vi "sha256_scram_client_final.vi"(9 "password":string, 10 "server_first_message":string, 11 "client_first_message":string) -> (3 "client_final_message":string)   [LabVIEW 2019, in "hashlib.lvlib"]
doc: "Calculates the <b>SCRAM-SHA-256 FINAL CLIENT MESSAGE</b> to send to the server to validate authentication based on the <b>client_first_message</b>, the <b>server_first_message</b> and the original <b>password</b>.\n\nRFC 5802\n\nCreated by: Ryan Pacini"
uses:
  hashlib.lvlib
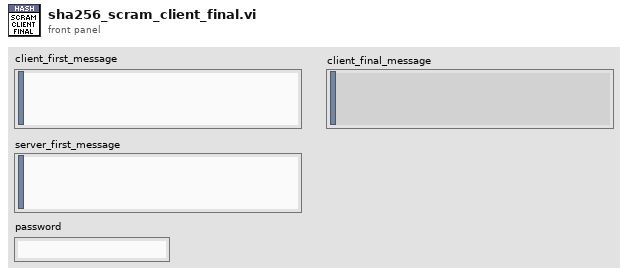
[diagram p1: front panel]
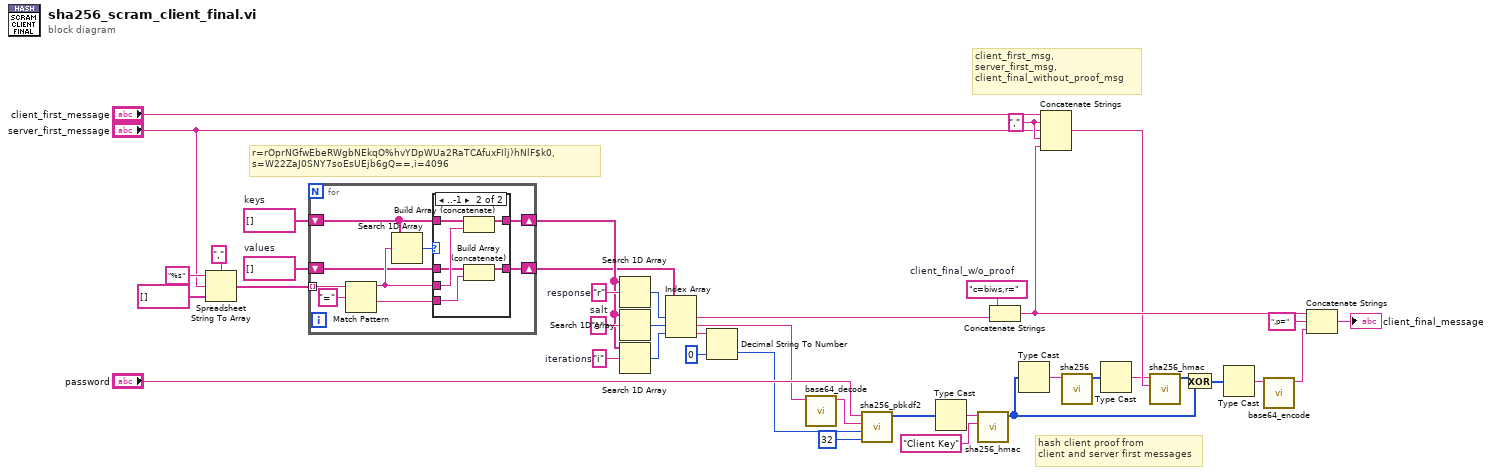
[diagram p0: block diagram]
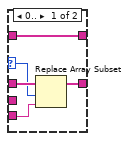
[diagram p2: hidden frame]
diagram:
  w3 = string[] []  # values
  w4 = string[] []  # keys
  w13 = "i"  # iterations
  w16 = "s"  # salt
  w17 = "r"  # response
  w34 = "," ("string")
  w33 = "c=biws,r="  # client_final_w/o_proof
  # "r=rOprNGfwEbeRWgbNEkqO%hvYDpWUa2RaTCAfuxFIlj)hNlF$k0,\ns=W22ZaJ0SNY7soEsUEjb6gQ==,i=4096"
  # "hash client proof from \nclient and server first messages"
  # "client_first_msg,\nserver_first_msg,\nclient_final_without_proof_msg"
  n1 = Spreadsheet String To Array(delimiter (Tab)=",", format string="%s", spreadsheet string="server_first_message", array type (2D Dbl)=string[] []) -> (array=w18:string[])
  n2 = for {
    tunnel: w18 -> [w50] mode=indexing
    shift-right: [w47] -> w2
    shift-left: w4 -> [w48]
    shift-right: [w43] -> w1
    shift-left: w3 -> [w44]
    n3 = Match Pattern(string=w50, regular expression="=") -> (before substring=w46:string, after substring=w42:string)  [unwired: 1 in, 2 out]
    n4 = Search 1D Array(1D array=w48, element=w46) -> (index of element=w45:i32)  [unwired: 1 in]
    n5 = case shown="..-1" w45 {
      selector: w45 -> [w52 _]
      tunnel: w48 -> [w55 w61]
      tunnel: [w55 w60] -> w47
      tunnel: w46 -> [_ w59]
      tunnel: w44 -> [w54 w58]
      tunnel: [w53 w57] -> w43
      tunnel: w42 -> [w51 w56]
      frame 0.. {
        n6 = Replace Array Subset(array=w54, new element=w51, index=w52) -> (w53:string[])
      }
      frame ..-1 {
        n7 = Build Array (concatenate)(w61, w59) -> (w60:string[])
        n8 = Build Array (concatenate)(w58, w56) -> (w57:string[])
      }
    }
  }
  n9 = Search 1D Array(1D array=w2, element=w17) -> (index of element=w15:i32)  [unwired: 1 in]
  n10 = Search 1D Array(1D array=w2, element=w16) -> (index of element=w14:i32)  [unwired: 1 in]
  n11 = Search 1D Array(1D array=w2, element=w13) -> (index of element=w12:i32)  [unwired: 1 in]
  n12 = Index Array(array=w1, index #1=w15, index #2=w14, index #3=w12) -> (element #1=w8:string, element #2=w7:string, element #3=w11:string)
  n13 = Decimal String To Number(string=w11, default (0L)=0 ("default (0 I32)")) -> (number=w6:i32)  [unwired: 1 in, 1 out]
  n14 = call "base64_decode.vi"("base64"=w7) -> ("string"=w21:string)  [unwired: 10 in]
  n15 = call "sha256_pbkdf2.vi"("dkLen (32octets=sha256)"=32 ("32octets=sha256"), "iterations"=w6, "salt"=w21, "password"="password") -> ("sha-256"=w29:u32[])  [unwired: 7 in]
  n16 = Type Cast(x=w29) -> (*(type *) &x=w31:string)  [unwired: 1 in]
  n17 = call "sha256_hmac.vi"("data"="Client Key" ("key"), "key"=w31) -> ("sha256"=w25:u32[])  [unwired: 9 in]
  n18 = Concatenate Strings(w33, w8) -> (w38:string)
  n19 = Type Cast(x=w25) -> (*(type *) &x=w22:string)  [unwired: 1 in]
  n20 = Concatenate Strings("client_first_message", w34, "server_first_message", w34, w38) -> (w35:string)
  n21 = call "sha256.vi"("data"=w22) -> ("sha256"=w23:u32[])  [unwired: 10 in]
  n22 = Type Cast(x=w23) -> (*(type *) &x=w30:string)  [unwired: 1 in]
  n23 = call "sha256_hmac.vi"("data"=w35, "key"=w30) -> ("sha256"=w24:u32[])  [unwired: 9 in]
  n24 = Exclusive Or(1:w25, 2:w24) -> (0:w26:u32[])
  n25 = Type Cast(x=w26) -> (*(type *) &x=w27:string)  [unwired: 1 in]
  n26 = call "base64_encode.vi"("string"=w27) -> ("base64"=w40:string)  [unwired: 10 in]
  n27 = Concatenate Strings(w38, ",p=", w40) -> (→"client_final_message":string)
